vi "CRYSelect Changed Name.vi"(7 "Option":string, 8 "Ref Data":string, 9 "Inserted Name":string[](array[string]), 10 "Origin Name":string[](array[string]), 11 "Type":string[](array[string])) -> (0 "Wave":T1, 1 "Result":T1, 2 "Value":T1, 3 "Cuve":T1)   [LabVIEW 2013]
uses:
  CRYSystem/Typedef Control/CRYChanged Data Array Cluster.ctl
  CRYSystem/Typedef Control/CRYChanged Data Cluster.ctl
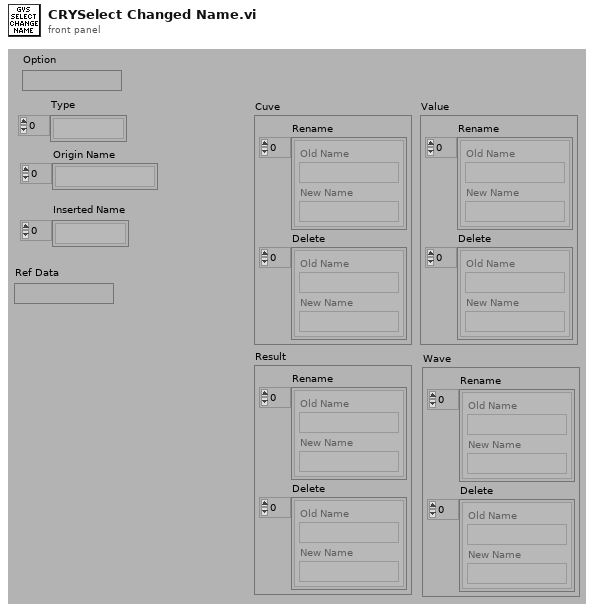
[diagram p1: front panel]
types:
  T1 = typedef "CRYChanged Data Array Cluster.ctl" = cluster{"Rename":T2[], "Delete":T2[]}
  T2 = typedef "CRYChanged Data Cluster.ctl" = cluster{"Old Name":string, "New Name":string}
  T3 = cluster{"CurveValue":string[], "Result":string[]}
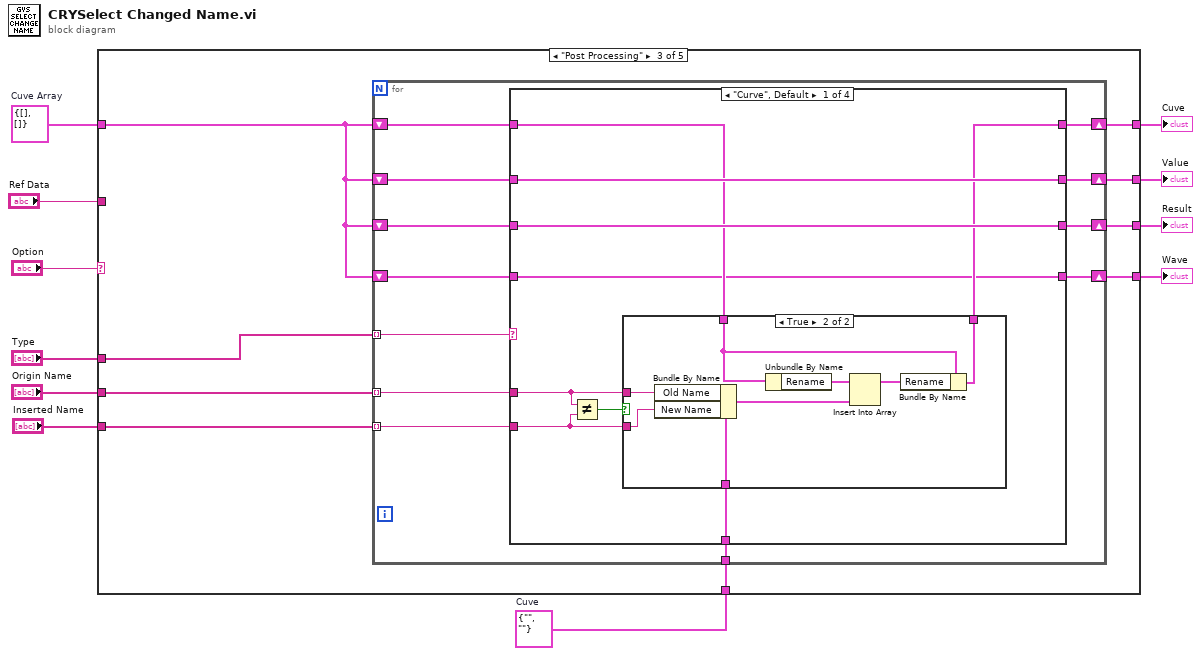
[diagram p0: block diagram]
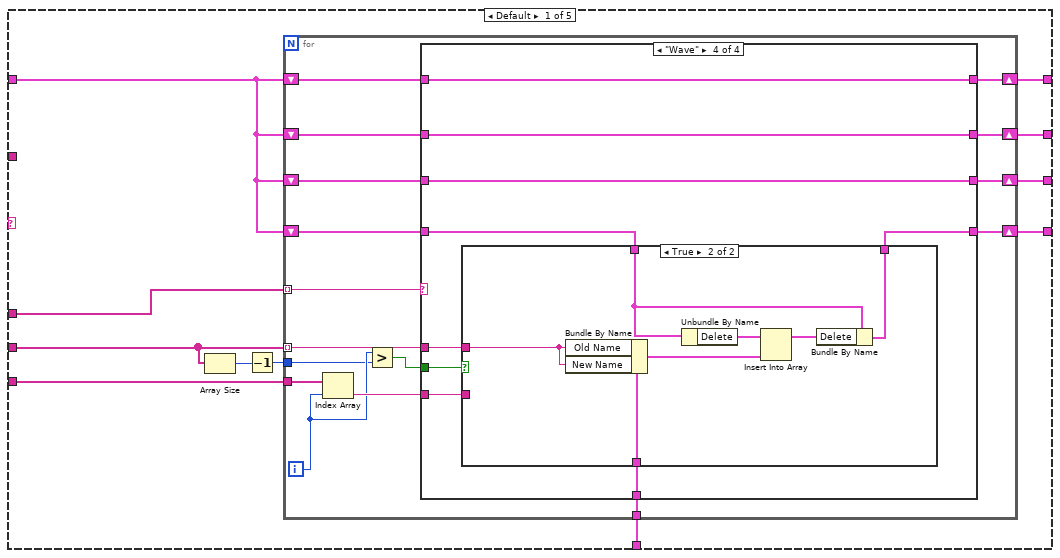
[diagram p2: hidden frame]
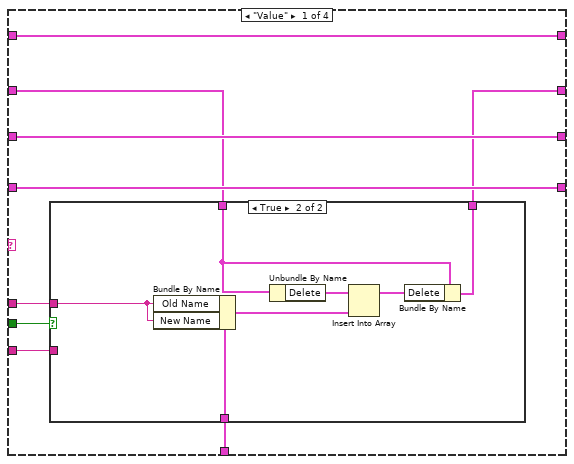
[diagram p3: hidden frame]
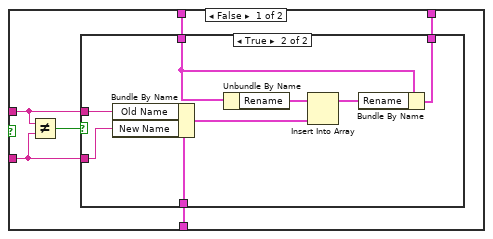
[diagram p4: hidden frame]
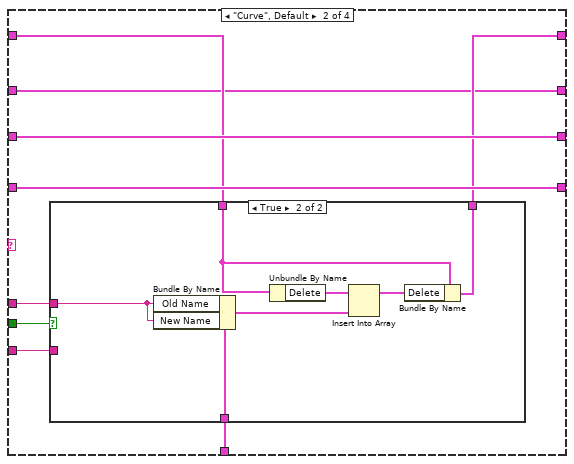
[diagram p6: hidden frame]
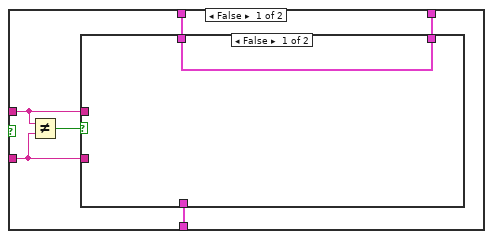
[diagram p7: hidden frame]
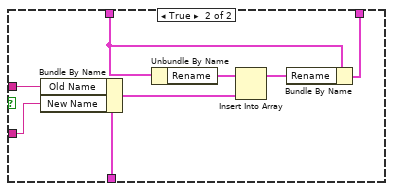
[diagram p8: hidden frame]
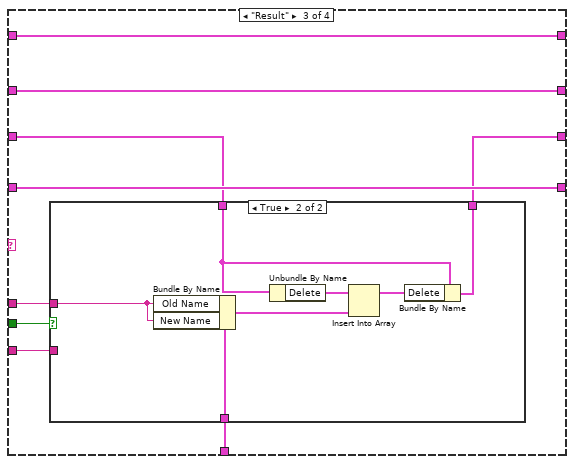
[diagram p9: hidden frame]
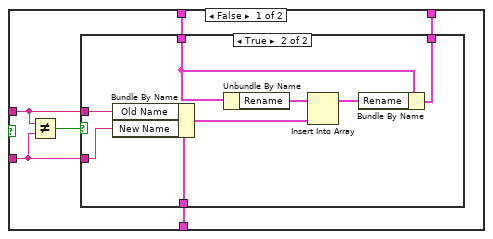
[diagram p10: hidden frame]
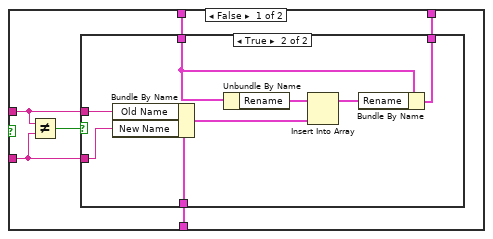
[diagram p12: hidden frame]
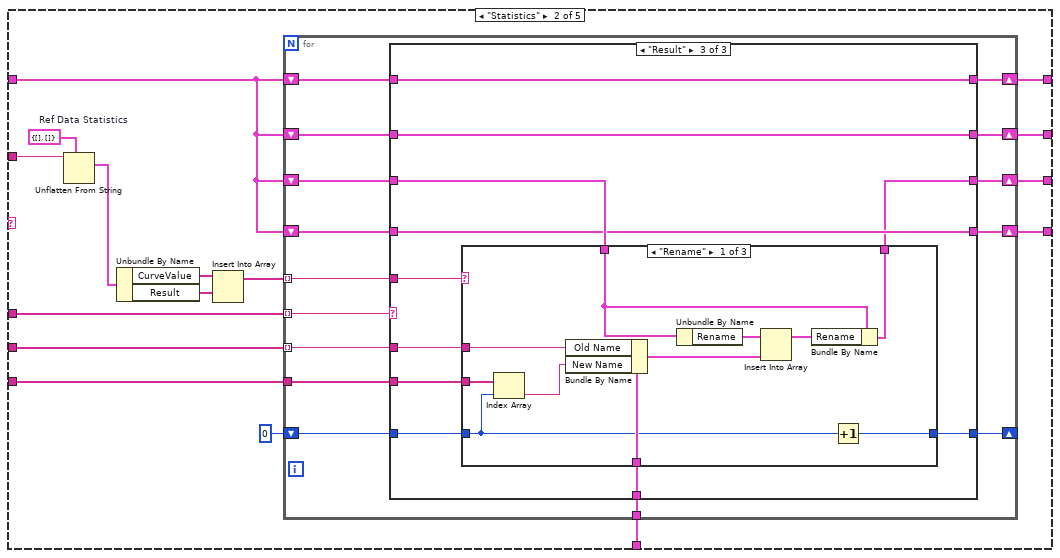
[diagram p14: hidden frame]
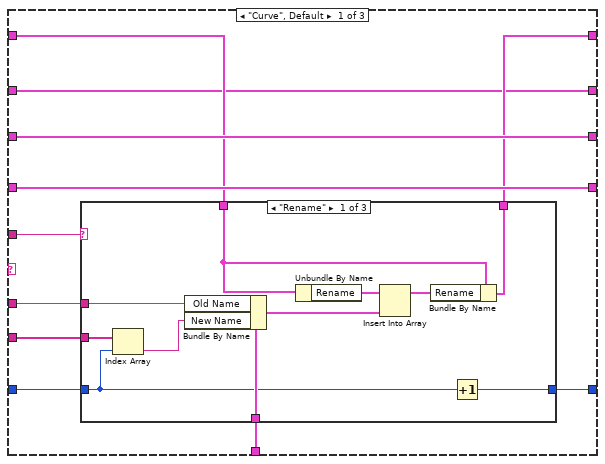
[diagram p15: hidden frame]
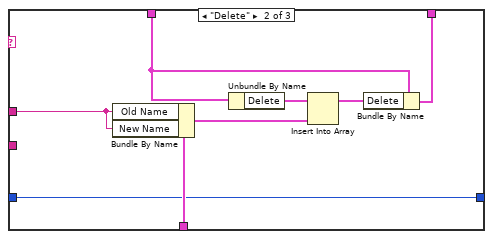
[diagram p16: hidden frame]
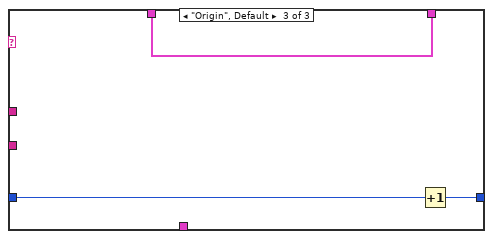
[diagram p17: hidden frame]
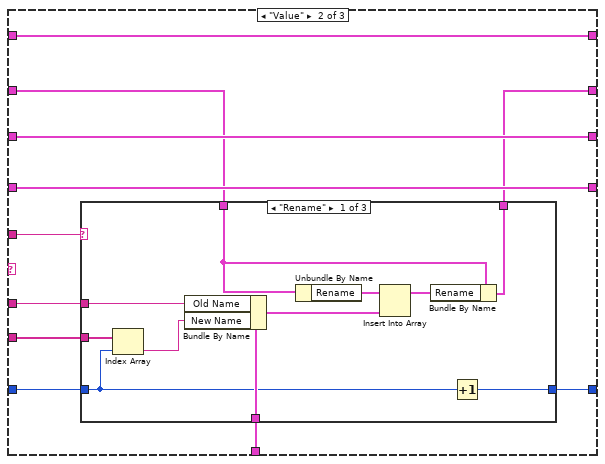
[diagram p18: hidden frame]
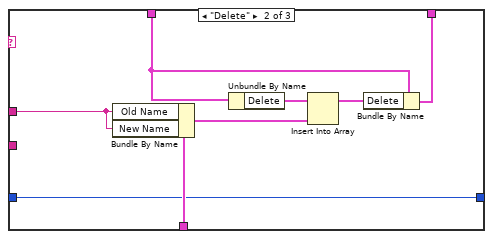
[diagram p19: hidden frame]
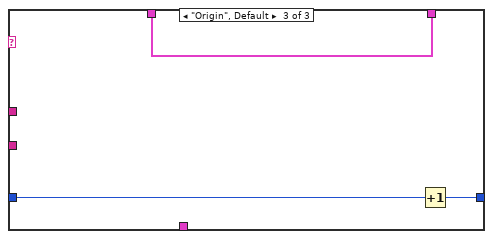
[diagram p20: hidden frame]
diagram:
  w6 = T1 {"Rename"=[], "Delete"=[]}  # Cuve Array
  w11 = T2 {"Old Name"="", "New Name"=""}  # Cuve
  n1 = case shown="\"Post Processing\"" "Option" {
    tunnel: w11 -> [w22 w178 w301 w394 w452]
    tunnel: [w21 w177 w300 w393 w454] -> w10
    tunnel: [w20 w176 w299 w392 w454] -> w9
    tunnel: [w19 w175 w298 w391 w454] -> w8
    tunnel: [w18 w174 w297 w390 w453] -> w7
    tunnel: w6 -> [w15 w173 w296 w389 w454]
    tunnel: "Origin Name" -> [w14 w172 w295 w388 w457]
    tunnel: "Inserted Name" -> [w13 w171 w294 w387 w455]
    tunnel: "Type" -> [w12 w170 w293 w386 _]
    tunnel: "Ref Data" -> [_ w167 _ _ w459]
    frame Default {
      n2 = Array Size(array=w14) -> (size(s)=w17:i32)
      n3 = Decrement(x=w17) -> (x-1=w16:i32)
      n4 = for {
        tunnel: w12 -> [w38] mode=indexing
        tunnel: w14 -> [w35] mode=indexing
        tunnel: w13 -> [w27]
        shift-right: [w36] -> w21
        shift-left: w15 -> [w37]
        tunnel: w22 -> [w34]
        shift-right: [w33] -> w20
        shift-left: w15 -> [w32]
        shift-right: [w31] -> w19
        shift-left: w15 -> [w30]
        shift-right: [w29] -> w18
        shift-left: w15 -> [w28]
        tunnel: w16 -> [w23]
        i -> [w24]
        n5 = Index Array(array=w27, index=w24) -> (element=w26:string)
        n6 = Greater?(x=w24, y=w23) -> (0:w25:bool)
        n7 = case shown="\"Wave\"" w38 {
          tunnel: w37 -> [w39 w72 w101 w132]
          tunnel: [w39 w71 w101 w132] -> w36
          tunnel: w35 -> [w43 w74 w105 w136]
          tunnel: w26 -> [w44 w75 w106 w137]
          tunnel: w34 -> [w47 w78 w109 w140]
          tunnel: [w40 w70 w108 w139] -> w33
          tunnel: w32 -> [w41 w70 w108 w139]
          tunnel: [w46 w77 w102 w138] -> w31
          tunnel: w30 -> [w46 w77 w103 w138]
          tunnel: [w45 w76 w107 w133] -> w29
          tunnel: w28 -> [w45 w76 w107 w134]
          tunnel: w25 -> [w42 w73 w104 w135]
          frame "Value" {
            n8 = case shown="True" w42 {
              tunnel: w41 -> [w53 w69]
              tunnel: [w52 w68] -> w40
              tunnel: w47 -> [w51 w67]
              tunnel: w44 -> [w50 _]
              tunnel: w43 -> [w49 w63]
              frame False {
                n9 = Not Equal?(x=w49, y=w50) -> (x != y?=w48:bool)
                n10 = case shown="True" w48 {
                  tunnel: w53 -> [w54 w59]
                  tunnel: [w54 w58] -> w52
                  tunnel: w51 -> [_ w62]
                  tunnel: w50 -> [_ w61]
                  tunnel: w49 -> [_ w60]
                  frame False {
                  }
                  frame True {
                    n11 = Bundle By Name(cluster=w62, "Old Name"=w60, "New Name"=w61) -> (w55:T2)
                    n12 = Unbundle By Name(w59) -> ("Rename"=w57:T2[])
                    n13 = Insert Into Array(array=w57, new element=w55) -> (w56:T2[])  [unwired: 1 in]
                    n14 = Bundle By Name(cluster=w59, "Rename"=w56) -> (w58:T1)
                  }
                }
              }
              frame True {
                n15 = Bundle By Name(cluster=w67, "Old Name"=w63, "New Name"=w63) -> (w64:T2)
                n16 = Unbundle By Name(w69) -> ("Delete"=w66:T2[])
                n17 = Insert Into Array(array=w66, new element=w64) -> (w65:T2[])  [unwired: 1 in]
                n18 = Bundle By Name(cluster=w69, "Delete"=w65) -> (w68:T1)
              }
            }
          }
          frame "Curve", Default {
            n19 = case shown="True" w73 {
              tunnel: w72 -> [w84 w100]
              tunnel: [w83 w99] -> w71
              tunnel: w78 -> [w82 w98]
              tunnel: w75 -> [w81 _]
              tunnel: w74 -> [w80 w94]
              frame False {
                n20 = Not Equal?(x=w80, y=w81) -> (x != y?=w79:bool)
                n21 = case shown="False" w79 {
                  tunnel: w84 -> [w85 w90]
                  tunnel: [w85 w89] -> w83
                  tunnel: w82 -> [_ w93]
                  tunnel: w81 -> [_ w92]
                  tunnel: w80 -> [_ w91]
                  frame False {
                  }
                  frame True {
                    n22 = Bundle By Name(cluster=w93, "Old Name"=w91, "New Name"=w92) -> (w86:T2)
                    n23 = Unbundle By Name(w90) -> ("Rename"=w88:T2[])
                    n24 = Insert Into Array(array=w88, new element=w86) -> (w87:T2[])  [unwired: 1 in]
                    n25 = Bundle By Name(cluster=w90, "Rename"=w87) -> (w89:T1)
                  }
                }
              }
              frame True {
                n26 = Bundle By Name(cluster=w98, "Old Name"=w94, "New Name"=w94) -> (w95:T2)
                n27 = Unbundle By Name(w100) -> ("Delete"=w97:T2[])
                n28 = Insert Into Array(array=w97, new element=w95) -> (w96:T2[])  [unwired: 1 in]
                n29 = Bundle By Name(cluster=w100, "Delete"=w96) -> (w99:T1)
              }
            }
          }
          frame "Result" {
            n30 = case shown="True" w104 {
              tunnel: w103 -> [w115 w131]
              tunnel: [w114 w130] -> w102
              tunnel: w109 -> [w113 w129]
              tunnel: w106 -> [w112 _]
              tunnel: w105 -> [w111 w125]
              frame False {
                n31 = Not Equal?(x=w111, y=w112) -> (x != y?=w110:bool)
                n32 = case shown="True" w110 {
                  tunnel: w115 -> [w116 w121]
                  tunnel: [w116 w120] -> w114
                  tunnel: w113 -> [_ w124]
                  tunnel: w112 -> [_ w123]
                  tunnel: w111 -> [_ w122]
                  frame False {
                  }
                  frame True {
                    n33 = Bundle By Name(cluster=w124, "Old Name"=w122, "New Name"=w123) -> (w117:T2)
                    n34 = Unbundle By Name(w121) -> ("Rename"=w119:T2[])
                    n35 = Insert Into Array(array=w119, new element=w117) -> (w118:T2[])  [unwired: 1 in]
                    n36 = Bundle By Name(cluster=w121, "Rename"=w118) -> (w120:T1)
                  }
                }
              }
              frame True {
                n37 = Bundle By Name(cluster=w129, "Old Name"=w125, "New Name"=w125) -> (w126:T2)
                n38 = Unbundle By Name(w131) -> ("Delete"=w128:T2[])
                n39 = Insert Into Array(array=w128, new element=w126) -> (w127:T2[])  [unwired: 1 in]
                n40 = Bundle By Name(cluster=w131, "Delete"=w127) -> (w130:T1)
              }
            }
          }
          frame "Wave" {
            n41 = case shown="True" w135 {
              tunnel: w134 -> [w146 w162]
              tunnel: [w145 w161] -> w133
              tunnel: w140 -> [w144 w160]
              tunnel: w137 -> [w143 _]
              tunnel: w136 -> [w142 w156]
              frame False {
                n42 = Not Equal?(x=w142, y=w143) -> (x != y?=w141:bool)
                n43 = case shown="True" w141 {
                  tunnel: w146 -> [w147 w152]
                  tunnel: [w147 w151] -> w145
                  tunnel: w144 -> [_ w155]
                  tunnel: w143 -> [_ w154]
                  tunnel: w142 -> [_ w153]
                  frame False {
                  }
                  frame True {
                    n44 = Bundle By Name(cluster=w155, "Old Name"=w153, "New Name"=w154) -> (w148:T2)
                    n45 = Unbundle By Name(w152) -> ("Rename"=w150:T2[])
                    n46 = Insert Into Array(array=w150, new element=w148) -> (w149:T2[])  [unwired: 1 in]
                    n47 = Bundle By Name(cluster=w152, "Rename"=w149) -> (w151:T1)
                  }
                }
              }
              frame True {
                n48 = Bundle By Name(cluster=w160, "Old Name"=w156, "New Name"=w156) -> (w157:T2)
                n49 = Unbundle By Name(w162) -> ("Delete"=w159:T2[])
                n50 = Insert Into Array(array=w159, new element=w157) -> (w158:T2[])  [unwired: 1 in]
                n51 = Bundle By Name(cluster=w162, "Delete"=w158) -> (w161:T1)
              }
            }
          }
        }
      }
    }
    frame "Statistics" {
      w169 = T3 {"CurveValue"=[], "Result"=[]}  # Ref Data Statistics
      n52 = Unflatten From String(type=w169, binary string=w167) -> (value=w168:T3)  [unwired: 3 in, 2 out]
      n53 = Unbundle By Name(w168) -> ("CurveValue"=w166:string[], "Result"=w165:string[])
      n54 = Insert Into Array(array=w166, new element=w165) -> (w164:string[])  [unwired: 1 in]
      n55 = for {
        tunnel: w170 -> [w193] mode=indexing
        tunnel: w172 -> [w190] mode=indexing
        tunnel: w171 -> [w179]
        shift-right: [w191] -> w177
        shift-left: w173 -> [w192]
        tunnel: w178 -> [w189]
        shift-right: [w188] -> w176
        shift-left: w173 -> [w187]
        shift-right: [w186] -> w175
        shift-left: w173 -> [w185]
        shift-right: [w184] -> w174
        shift-left: w173 -> [w183]
        tunnel: w164 -> [w182] mode=indexing
        shift-right: [w181] -> _
        shift-left: 0 -> [w180]
        n56 = case shown="\"Result\"" w193 {
          tunnel: w192 -> [w200 w229 w263]
          tunnel: [w199 w229 w263] -> w191
          tunnel: w190 -> [w201 w234 w269]
          tunnel: w189 -> [w204 w237 w270]
          tunnel: [w198 w227 w268] -> w188
          tunnel: w187 -> [w198 w228 w268]
          tunnel: [w203 w236 w260] -> w186
          tunnel: w185 -> [w203 w236 w262]
          tunnel: [w202 w235 w261] -> w184
          tunnel: w183 -> [w202 w235 w261]
          tunnel: w182 -> [w197 w233 w267]
          tunnel: [w196 w232 w266] -> w181
          tunnel: w180 -> [w195 w231 w265]
          tunnel: w179 -> [w194 w230 w264]
          frame "Curve", Default {
            n57 = case shown="\"Rename\"" w197 {
              tunnel: w200 -> [w215 w223 w226]
              tunnel: [w214 w222 w226] -> w199
              tunnel: w204 -> [w213 w221 _]
              tunnel: w201 -> [w212 w217 _]
              tunnel: [w208 w216 w224] -> w196
              tunnel: w195 -> [w205 w216 w225]
              tunnel: w194 -> [w207 _ _]
              frame "Rename" {
                n58 = Index Array(array=w207, index=w205) -> (element=w206:string)
                n59 = Bundle By Name(cluster=w213, "Old Name"=w212, "New Name"=w206) -> (w209:T2)
                n60 = Unbundle By Name(w215) -> ("Rename"=w211:T2[])
                n61 = Insert Into Array(array=w211, new element=w209) -> (w210:T2[])  [unwired: 1 in]
                n62 = Bundle By Name(cluster=w215, "Rename"=w210) -> (w214:T1)
                n63 = Increment(x=w205) -> (x+1=w208:i32)
              }
              frame "Delete" {
                n64 = Bundle By Name(cluster=w221, "Old Name"=w217, "New Name"=w217) -> (w218:T2)
                n65 = Unbundle By Name(w223) -> ("Delete"=w220:T2[])
                n66 = Insert Into Array(array=w220, new element=w218) -> (w219:T2[])  [unwired: 1 in]
                n67 = Bundle By Name(cluster=w223, "Delete"=w219) -> (w222:T1)
              }
              frame "Origin", Default {
                n68 = Increment(x=w225) -> (x+1=w224:i32)
              }
            }
          }
          frame "Value" {
            n69 = case shown="\"Rename\"" w233 {
              tunnel: w228 -> [w248 w256 w259]
              tunnel: [w247 w255 w259] -> w227
              tunnel: w237 -> [w246 w254 _]
              tunnel: w234 -> [w245 w250 _]
              tunnel: [w241 w249 w257] -> w232
              tunnel: w231 -> [w238 w249 w258]
              tunnel: w230 -> [w240 _ _]
              frame "Rename" {
                n70 = Index Array(array=w240, index=w238) -> (element=w239:string)
                n71 = Bundle By Name(cluster=w246, "Old Name"=w245, "New Name"=w239) -> (w242:T2)
                n72 = Unbundle By Name(w248) -> ("Rename"=w244:T2[])
                n73 = Insert Into Array(array=w244, new element=w242) -> (w243:T2[])  [unwired: 1 in]
                n74 = Bundle By Name(cluster=w248, "Rename"=w243) -> (w247:T1)
                n75 = Increment(x=w238) -> (x+1=w241:i32)
              }
              frame "Delete" {
                n76 = Bundle By Name(cluster=w254, "Old Name"=w250, "New Name"=w250) -> (w251:T2)
                n77 = Unbundle By Name(w256) -> ("Delete"=w253:T2[])
                n78 = Insert Into Array(array=w253, new element=w251) -> (w252:T2[])  [unwired: 1 in]
                n79 = Bundle By Name(cluster=w256, "Delete"=w252) -> (w255:T1)
              }
              frame "Origin", Default {
                n80 = Increment(x=w258) -> (x+1=w257:i32)
              }
            }
          }
          frame "Result" {
            n81 = case shown="\"Rename\"" w267 {
              tunnel: w262 -> [w281 w289 w292]
              tunnel: [w280 w288 w292] -> w260
              tunnel: w270 -> [w279 w287 _]
              tunnel: w269 -> [w278 w283 _]
              tunnel: [w274 w282 w290] -> w266
              tunnel: w265 -> [w271 w282 w291]
              tunnel: w264 -> [w273 _ _]
              frame "Rename" {
                n82 = Index Array(array=w273, index=w271) -> (element=w272:string)
                n83 = Bundle By Name(cluster=w279, "Old Name"=w278, "New Name"=w272) -> (w275:T2)
                n84 = Unbundle By Name(w281) -> ("Rename"=w277:T2[])
                n85 = Insert Into Array(array=w277, new element=w275) -> (w276:T2[])  [unwired: 1 in]
                n86 = Bundle By Name(cluster=w281, "Rename"=w276) -> (w280:T1)
                n87 = Increment(x=w271) -> (x+1=w274:i32)
              }
              frame "Delete" {
                n88 = Bundle By Name(cluster=w287, "Old Name"=w283, "New Name"=w283) -> (w284:T2)
                n89 = Unbundle By Name(w289) -> ("Delete"=w286:T2[])
                n90 = Insert Into Array(array=w286, new element=w284) -> (w285:T2[])  [unwired: 1 in]
                n91 = Bundle By Name(cluster=w289, "Delete"=w285) -> (w288:T1)
              }
              frame "Origin", Default {
                n92 = Increment(x=w291) -> (x+1=w290:i32)
              }
            }
          }
        }
      }
    }
    frame "Post Processing" {
      n93 = for {
        tunnel: w293 -> [w313] mode=indexing
        tunnel: w295 -> [w310] mode=indexing
        tunnel: w294 -> [w302] mode=indexing
        shift-right: [w311] -> w300
        shift-left: w296 -> [w312]
        tunnel: w301 -> [w309]
        shift-right: [w308] -> w299
        shift-left: w296 -> [w307]
        shift-right: [w306] -> w298
        shift-left: w296 -> [w305]
        shift-right: [w304] -> w297
        shift-left: w296 -> [w303]
        n94 = case shown="\"Curve\", Default" w313 {
          tunnel: w312 -> [w316 w337 w355 w370]
          tunnel: [w315 w337 w355 w370] -> w311
          tunnel: w310 -> [w319 w338 w356 w373]
          tunnel: w309 -> [w322 w340 w358 w376]
          tunnel: [w321 w333 w357 w375] -> w308
          tunnel: w307 -> [w321 w334 w357 w375]
          tunnel: [w320 w339 w351 w374] -> w306
          tunnel: w305 -> [w320 w339 w352 w374]
          tunnel: [w314 w332 w350 w371] -> w304
          tunnel: w303 -> [w314 w332 w350 w372]
          tunnel: w302 -> [w317 w335 w353 w368]
          frame "Curve", Default {
            n95 = Not Equal?(x=w319, y=w317) -> (x != y?=w318:bool)
            n96 = case shown="True" w318 {
              tunnel: w316 -> [w323 w329]
              tunnel: [w323 w328] -> w315
              tunnel: w322 -> [_ w331]
              tunnel: w319 -> [_ w330]
              tunnel: w317 -> [_ w324]
              frame False {
              }
              frame True {
                n97 = Bundle By Name(cluster=w331, "Old Name"=w330, "New Name"=w324) -> (w325:T2)
                n98 = Unbundle By Name(w329) -> ("Rename"=w327:T2[])
                n99 = Insert Into Array(array=w327, new element=w325) -> (w326:T2[])  [unwired: 1 in]
                n100 = Bundle By Name(cluster=w329, "Rename"=w326) -> (w328:T1)
              }
            }
          }
          frame "Value" {
            n101 = Not Equal?(x=w338, y=w335) -> (x != y?=w336:bool)
            n102 = case shown="True" w336 {
              tunnel: w334 -> [w341 w347]
              tunnel: [w341 w346] -> w333
              tunnel: w340 -> [_ w349]
              tunnel: w338 -> [_ w348]
              tunnel: w335 -> [_ w342]
              frame False {
              }
              frame True {
                n103 = Bundle By Name(cluster=w349, "Old Name"=w348, "New Name"=w342) -> (w343:T2)
                n104 = Unbundle By Name(w347) -> ("Rename"=w345:T2[])
                n105 = Insert Into Array(array=w345, new element=w343) -> (w344:T2[])  [unwired: 1 in]
                n106 = Bundle By Name(cluster=w347, "Rename"=w344) -> (w346:T1)
              }
            }
          }
          frame "Result" {
            n107 = Not Equal?(x=w356, y=w353) -> (x != y?=w354:bool)
            n108 = case shown="True" w354 {
              tunnel: w352 -> [w359 w365]
              tunnel: [w359 w364] -> w351
              tunnel: w358 -> [_ w367]
              tunnel: w356 -> [_ w366]
              tunnel: w353 -> [_ w360]
              frame False {
              }
              frame True {
                n109 = Bundle By Name(cluster=w367, "Old Name"=w366, "New Name"=w360) -> (w361:T2)
                n110 = Unbundle By Name(w365) -> ("Rename"=w363:T2[])
                n111 = Insert Into Array(array=w363, new element=w361) -> (w362:T2[])  [unwired: 1 in]
                n112 = Bundle By Name(cluster=w365, "Rename"=w362) -> (w364:T1)
              }
            }
          }
          frame "Wave" {
            n113 = Not Equal?(x=w373, y=w368) -> (x != y?=w369:bool)
            n114 = case shown="True" w369 {
              tunnel: w372 -> [w377 w383]
              tunnel: [w377 w382] -> w371
              tunnel: w376 -> [_ w385]
              tunnel: w373 -> [_ w384]
              tunnel: w368 -> [_ w378]
              frame False {
              }
              frame True {
                n115 = Bundle By Name(cluster=w385, "Old Name"=w384, "New Name"=w378) -> (w379:T2)
                n116 = Unbundle By Name(w383) -> ("Rename"=w381:T2[])
                n117 = Insert Into Array(array=w381, new element=w379) -> (w380:T2[])  [unwired: 1 in]
                n118 = Bundle By Name(cluster=w383, "Rename"=w380) -> (w382:T1)
              }
            }
          }
        }
      }
    }
    frame "Analysis" {
      n119 = for {
        tunnel: w386 -> [w406] mode=indexing
        tunnel: w388 -> [w403] mode=indexing
        tunnel: w387 -> [w395] mode=indexing
        shift-right: [w404] -> w393
        shift-left: w389 -> [w405]
        tunnel: w394 -> [w402]
        shift-right: [w401] -> w392
        shift-left: w389 -> [w400]
        shift-right: [w399] -> w391
        shift-left: w389 -> [w398]
        shift-right: [w397] -> w390
        shift-left: w389 -> [w396]
        n120 = case shown="\"Value\"" w406 {
          tunnel: w405 -> [w409 w425 w436 w444]
          tunnel: [w408 w425 w436 w444] -> w404
          tunnel: w403 -> [w414 w426 w437 w447]
          tunnel: w402 -> [w417 w428 w439 w450]
          tunnel: [w416 w419 w438 w449] -> w401
          tunnel: w400 -> [w416 w420 w438 w449]
          tunnel: [w415 w427 w430 w448] -> w399
          tunnel: w398 -> [w415 w427 w431 w448]
          tunnel: [w407 w418 w429 w445] -> w397
          tunnel: w396 -> [w407 w418 w429 w446]
          tunnel: w395 -> [w410 w421 w432 w440]
          frame "Curve", Default {
            n121 = Bundle By Name(cluster=w417, "Old Name"=w414, "New Name"=w410) -> (w411:T2)
            n122 = Unbundle By Name(w409) -> ("Rename"=w413:T2[])
            n123 = Insert Into Array(array=w413, new element=w411) -> (w412:T2[])  [unwired: 1 in]
            n124 = Bundle By Name(cluster=w409, "Rename"=w412) -> (w408:T1)
          }
          frame "Value" {
            n125 = Bundle By Name(cluster=w428, "Old Name"=w426, "New Name"=w421) -> (w422:T2)
            n126 = Unbundle By Name(w420) -> ("Rename"=w424:T2[])
            n127 = Insert Into Array(array=w424, new element=w422) -> (w423:T2[])  [unwired: 1 in]
            n128 = Bundle By Name(cluster=w420, "Rename"=w423) -> (w419:T1)
          }
          frame "Result" {
            n129 = Bundle By Name(cluster=w439, "Old Name"=w437, "New Name"=w432) -> (w433:T2)
            n130 = Unbundle By Name(w431) -> ("Rename"=w435:T2[])
            n131 = Insert Into Array(array=w435, new element=w433) -> (w434:T2[])  [unwired: 1 in]
            n132 = Bundle By Name(cluster=w431, "Rename"=w434) -> (w430:T1)
          }
          frame "Wave" {
            n133 = Bundle By Name(cluster=w450, "Old Name"=w447, "New Name"=w440) -> (w441:T2)
            n134 = Unbundle By Name(w446) -> ("Rename"=w443:T2[])
            n135 = Insert Into Array(array=w443, new element=w441) -> (w442:T2[])  [unwired: 1 in]
            n136 = Bundle By Name(cluster=w446, "Rename"=w442) -> (w445:T1)
          }
        }
      }
    }
    frame "Acquisition" {
      n137 = Unflatten From String(type=string[] [], binary string=w459) -> (value=w456:string[])  [unwired: 3 in, 2 out]
      n138 = for {
        tunnel: w457 -> [w461] mode=indexing
        tunnel: w456 -> [w467] mode=indexing
        tunnel: w455 -> [w460]
        shift-right: [w465] -> w453
        shift-left: w454 -> [w466]
        tunnel: w452 -> [w464]
        shift-right: [w463] -> _
        shift-left: 0 -> [w462]
        n139 = case shown="\"Rename\"" w467 {
          tunnel: w466 -> [w470 w478 w484]
          tunnel: [w470 w476 w485] -> w465
          tunnel: w464 -> [_ w477 w486]
          tunnel: [w468 w475 w483] -> w463
          tunnel: w462 -> [w469 w472 w483]
          tunnel: w461 -> [_ w474 w482]
          tunnel: w460 -> [_ w473 _]
          frame "Origin", Default {
            n140 = Increment(x=w469) -> (x+1=w468:i32)
          }
          frame "Rename" {
            n141 = Index Array(array=w473, index=w472) -> (element=w471:string)
            n142 = Bundle By Name(cluster=w477, "Old Name"=w474, "New Name"=w471) -> (w479:T2)
            n143 = Unbundle By Name(w478) -> ("Rename"=w481:T2[])
            n144 = Insert Into Array(array=w481, new element=w479) -> (w480:T2[])  [unwired: 1 in]
            n145 = Bundle By Name(cluster=w478, "Rename"=w480) -> (w476:T1)
            n146 = Increment(x=w472) -> (x+1=w475:i32)
          }
          frame "Delete" {
            n147 = Bundle By Name(cluster=w486, "Old Name"=w482, "New Name"=w482) -> (w489:T2)
            n148 = Unbundle By Name(w484) -> ("Delete"=w487:T2[])
            n149 = Insert Into Array(array=w487, new element=w489) -> (w488:T2[])  [unwired: 1 in]
            n150 = Bundle By Name(cluster=w484, "Delete"=w488) -> (w485:T1)
          }
        }
      }
    }
  }
  "Cuve" <- w10
  "Value" <- w9
  "Result" <- w8
  "Wave" <- w7
